vi "Int2Dbl.vi"(11 "AI_raw":i16) -> (3 "AI_converted [V]":dbl format="%#.6f")   [LabVIEW 2020, in "FPGA_IO.lvlib"]
doc: "Convert 12-bit AI integer values into floating point (DBL) values."
uses:
  FPGA_IO.lvlib
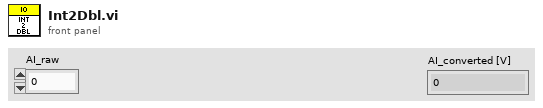
[diagram p1: front panel]
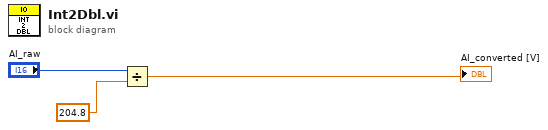
[diagram p0: block diagram]
diagram:
  n1 = Divide(x="AI_raw", y=204.8) -> (x/y=→"AI_converted [V]":dbl)
